vi "calc_Chi-CO2.vi"(0 "command parameter":T1={"CO2 ref"=392.0, "CO2 span"=372.0, "H2O ref"=0.0, "H2O span"=0.0, "Zi"=0.0, "Zt"=1.2, "Zm"=0.0, "S"=0.0, "Temp [C]"=50.0, "Pressure [hPa]"=135.0, "Licor-Sources"=["CO2A W", "CO2B W", "H2OA W", "H2OB W", "T C", "T V", "P kPa", "P V", "RH %", "CO2A um/m", "CO2B um/m", "H2OA mm/m", "H2OB mm/m"], "Licor-Pump"="Off", "Zeitstempel"=timestamp(0 s since 1904-01-01)} {"Pressure [hPa]" format="%_5g"; "Temp [C]" format="%.2f"; "CO2 ref" format="%.2f"; "CO2 span" format="%.2g"; "H2O ref" format="%.2g"; "H2O span" format="%.2g"; "Zt" format="%#_4g"}, 9 "Raw_CO2_A":dbl format="%#_13g", 11 "Raw_CO2_B":dbl format="%#_13g") -> (8 "Chi_CO2_B":dbl)   [LabVIEW 2010, in "Licor-Steuerung.lvlib"]
uses:
  Licor-Steuerung.lvlib
  control/Licor-Parameter.ctl
  LicorLI7000/conventions/Licor-Source.ctl
  control/Licor-Pump.ctl
  LicorLI7000/Z parameter.ctl
  LicorLI7000/conventions/Substance.ctl
  LicorLI7000/LicorLI7000.lvlib
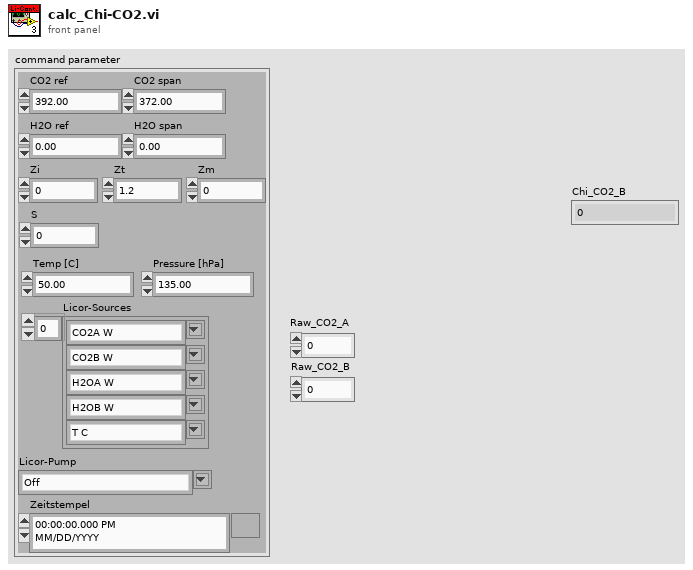
[diagram p1: front panel]
types:
  T1 = typedef "Licor-Steuerung.lvlib/Licor-Parameter.ctl" = cluster{"CO2 ref":dbl, "CO2 span":dbl, "H2O ref":dbl, "H2O span":dbl, "Zi":dbl, "Zt":dbl, "Zm":dbl, "S":dbl, "Temp [C]":dbl, "Pressure [hPa]":dbl, "Licor-Sources":T2[], "Licor-Pump":T3, "Zeitstempel":timestamp}
  T2 = typedef "LicorLI7000.lvlib/Licor-Source.ctl" = string
  T3 = typedef "Licor-Steuerung.lvlib/Licor-Pump.ctl" = string
  T4 = typedef "LicorLI7000.lvlib/Substance.ctl" = enum16{"CO2", "H2O"}
  T5 = typedef "LicorLI7000.lvlib/Z parameter.ctl" = cluster{"zi":dbl, "zt":dbl, "zm":dbl}
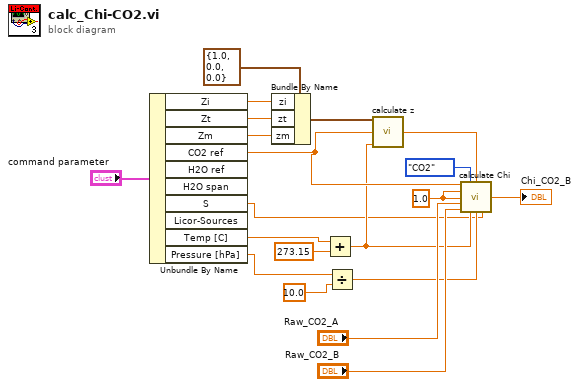
[diagram p0: block diagram]
diagram:
  w8 = 1.0 ("Psi_A")
  n1 = Unbundle By Name("command parameter") -> ("Zi"=w17:dbl, "Zt"=w16:dbl, "Zm"=w15:dbl, "CO2 ref"=w9:dbl, "S"=w2:dbl, "Temp [C]"=w13:dbl, "Pressure [hPa]"=w4:dbl)  [unwired: 3 out]
  n2 = Bundle By Name(cluster=T5 {"zi"=1.0, "zt"=0.0, "zm"=0.0} ("Z"), "zi"=w17, "zt"=w16, "zm"=w15) -> (w14:T5)
  n3 = Add(x=w13, y=273.15) -> (x+y=w5:dbl)
  n4 = Divide(x=w4, y=10.0) -> (x/y=w3:dbl)
  n5 = call "calculate z.vi"("Z"=w14, "Chi_A"=w9, "T [K]"=w5) -> ("Z"=w10:dbl)  [unwired: 12 in]
  n6 = call "calculate Chi.vi"("Chi_A"=w9, "CO2/H2O"=Substance."CO2", "Z"=w10, "Psi_A"=w8, "Psi_B"=w8, "W_A [raw signal]"="Raw_CO2_A", "W_B [raw signal]"="Raw_CO2_B", "T [K]"=w5, "P [kPa]"=w3, "S"=w2) -> ("Chi_B"=→"Chi_CO2_B":dbl)  [unwired: 5 in]
